vi "uc480_LiveStream_8bitAMb.vi"() -> ()   [LabVIEW 2013]
doc: "Capture_8bit nimmt kontinuierlich Bilder von der Kamera auf und zeigt diese an."
panel:
  out "Row sigma":dbl
  out "Col sigma":dbl
  out "Fits Graphs":cluster{i32[], "Best Gaussian Fit":dbl[]}[](graph)
  out "Row Cent":dbl
  out "Col Cent":dbl
  out "Col 1/e^2 rad":cluster{i32[], dbl[]}(graph)
  out "Row 1/e^2 rad":cluster{i32[], dbl[]}(graph)
  in  "Clip Threshold":dbl
  out "Col Centroid":cluster{i32[], dbl[]}[](graph)
  out "Row Centroid":cluster{i32[], dbl[]}[](graph)
  in  "Clear Charts":bool
  out "Centroid position":cluster{dbl[], dbl[]}(graph)
  out "Staturation":dbl(slide) scale=0.0..255.0
  out "Histogram":dynamicdata(graph)
  out "min value":u8
  out "max value":u8
  out "size(s)":i32[](array[numeric])
  out "output array":u8[][](array[numeric])
  out "error out":errorcluster caption="error"
  in  "Camera ID":u32
  in  "Frame rate":dbl(slide)=30.0 min=4.876716604244694 max=13.962044182888818 step=6.675e-05 scale=4.876716604244694..13.962044182888818 scale format="%^#_3g"
  in  "Pixel clock":i32(slide)=20 min=5 max=43 scale=5.0..43.0
  in  "Exposure time":dbl(slide)=33.21525 min=0.06675 max=71.556 step=0.06675 scale=0.06675..71.556 scale format="%#.3g"
  in  "Edge Filter":i32(ring)=2 items=["High"=1, "Low"=2]
  in  "Edge Filter Enable / Disable":bool
  in  "Blacklevel Offset":i32(slide) min=0 max=255 scale=0.0..255.0
  in  "Blacklevel compensation":bool
  in  "Hotpixel correction":bool
  in  "Master Gain":i32(slide) min=0 max=100 scale=0.0..100.0
  in  "Autogain":bool
  out "Height":i32=480
  out "Width":i32=640
  out "Bits/Pixel":i32=8
  out "FPS":dbl=6.258409738085552
  in  "Stopp":bool
  out "Video":u8[][](graph)
  # "Stop Program here"
  # "2 sigma = 1/e^2 (13.5%) radius\nFWHM = 2.35 sigma"
  # "Image information"
  # "Settings"
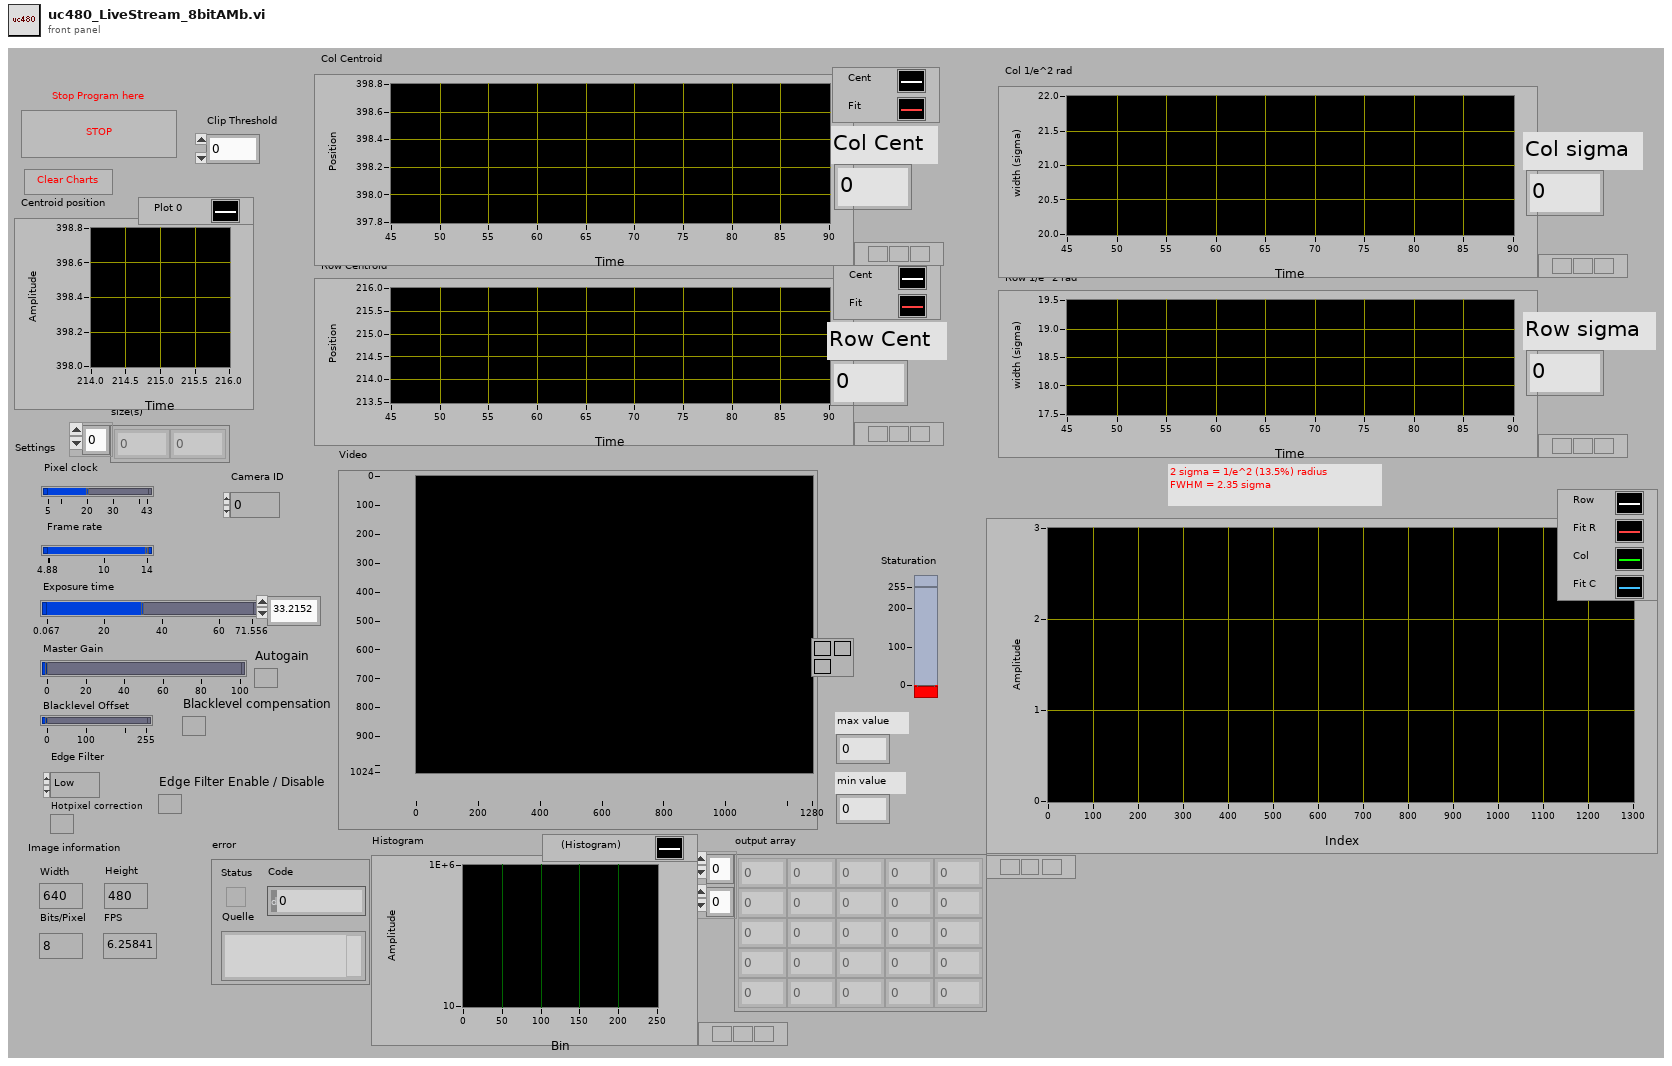
[diagram p1: front panel]
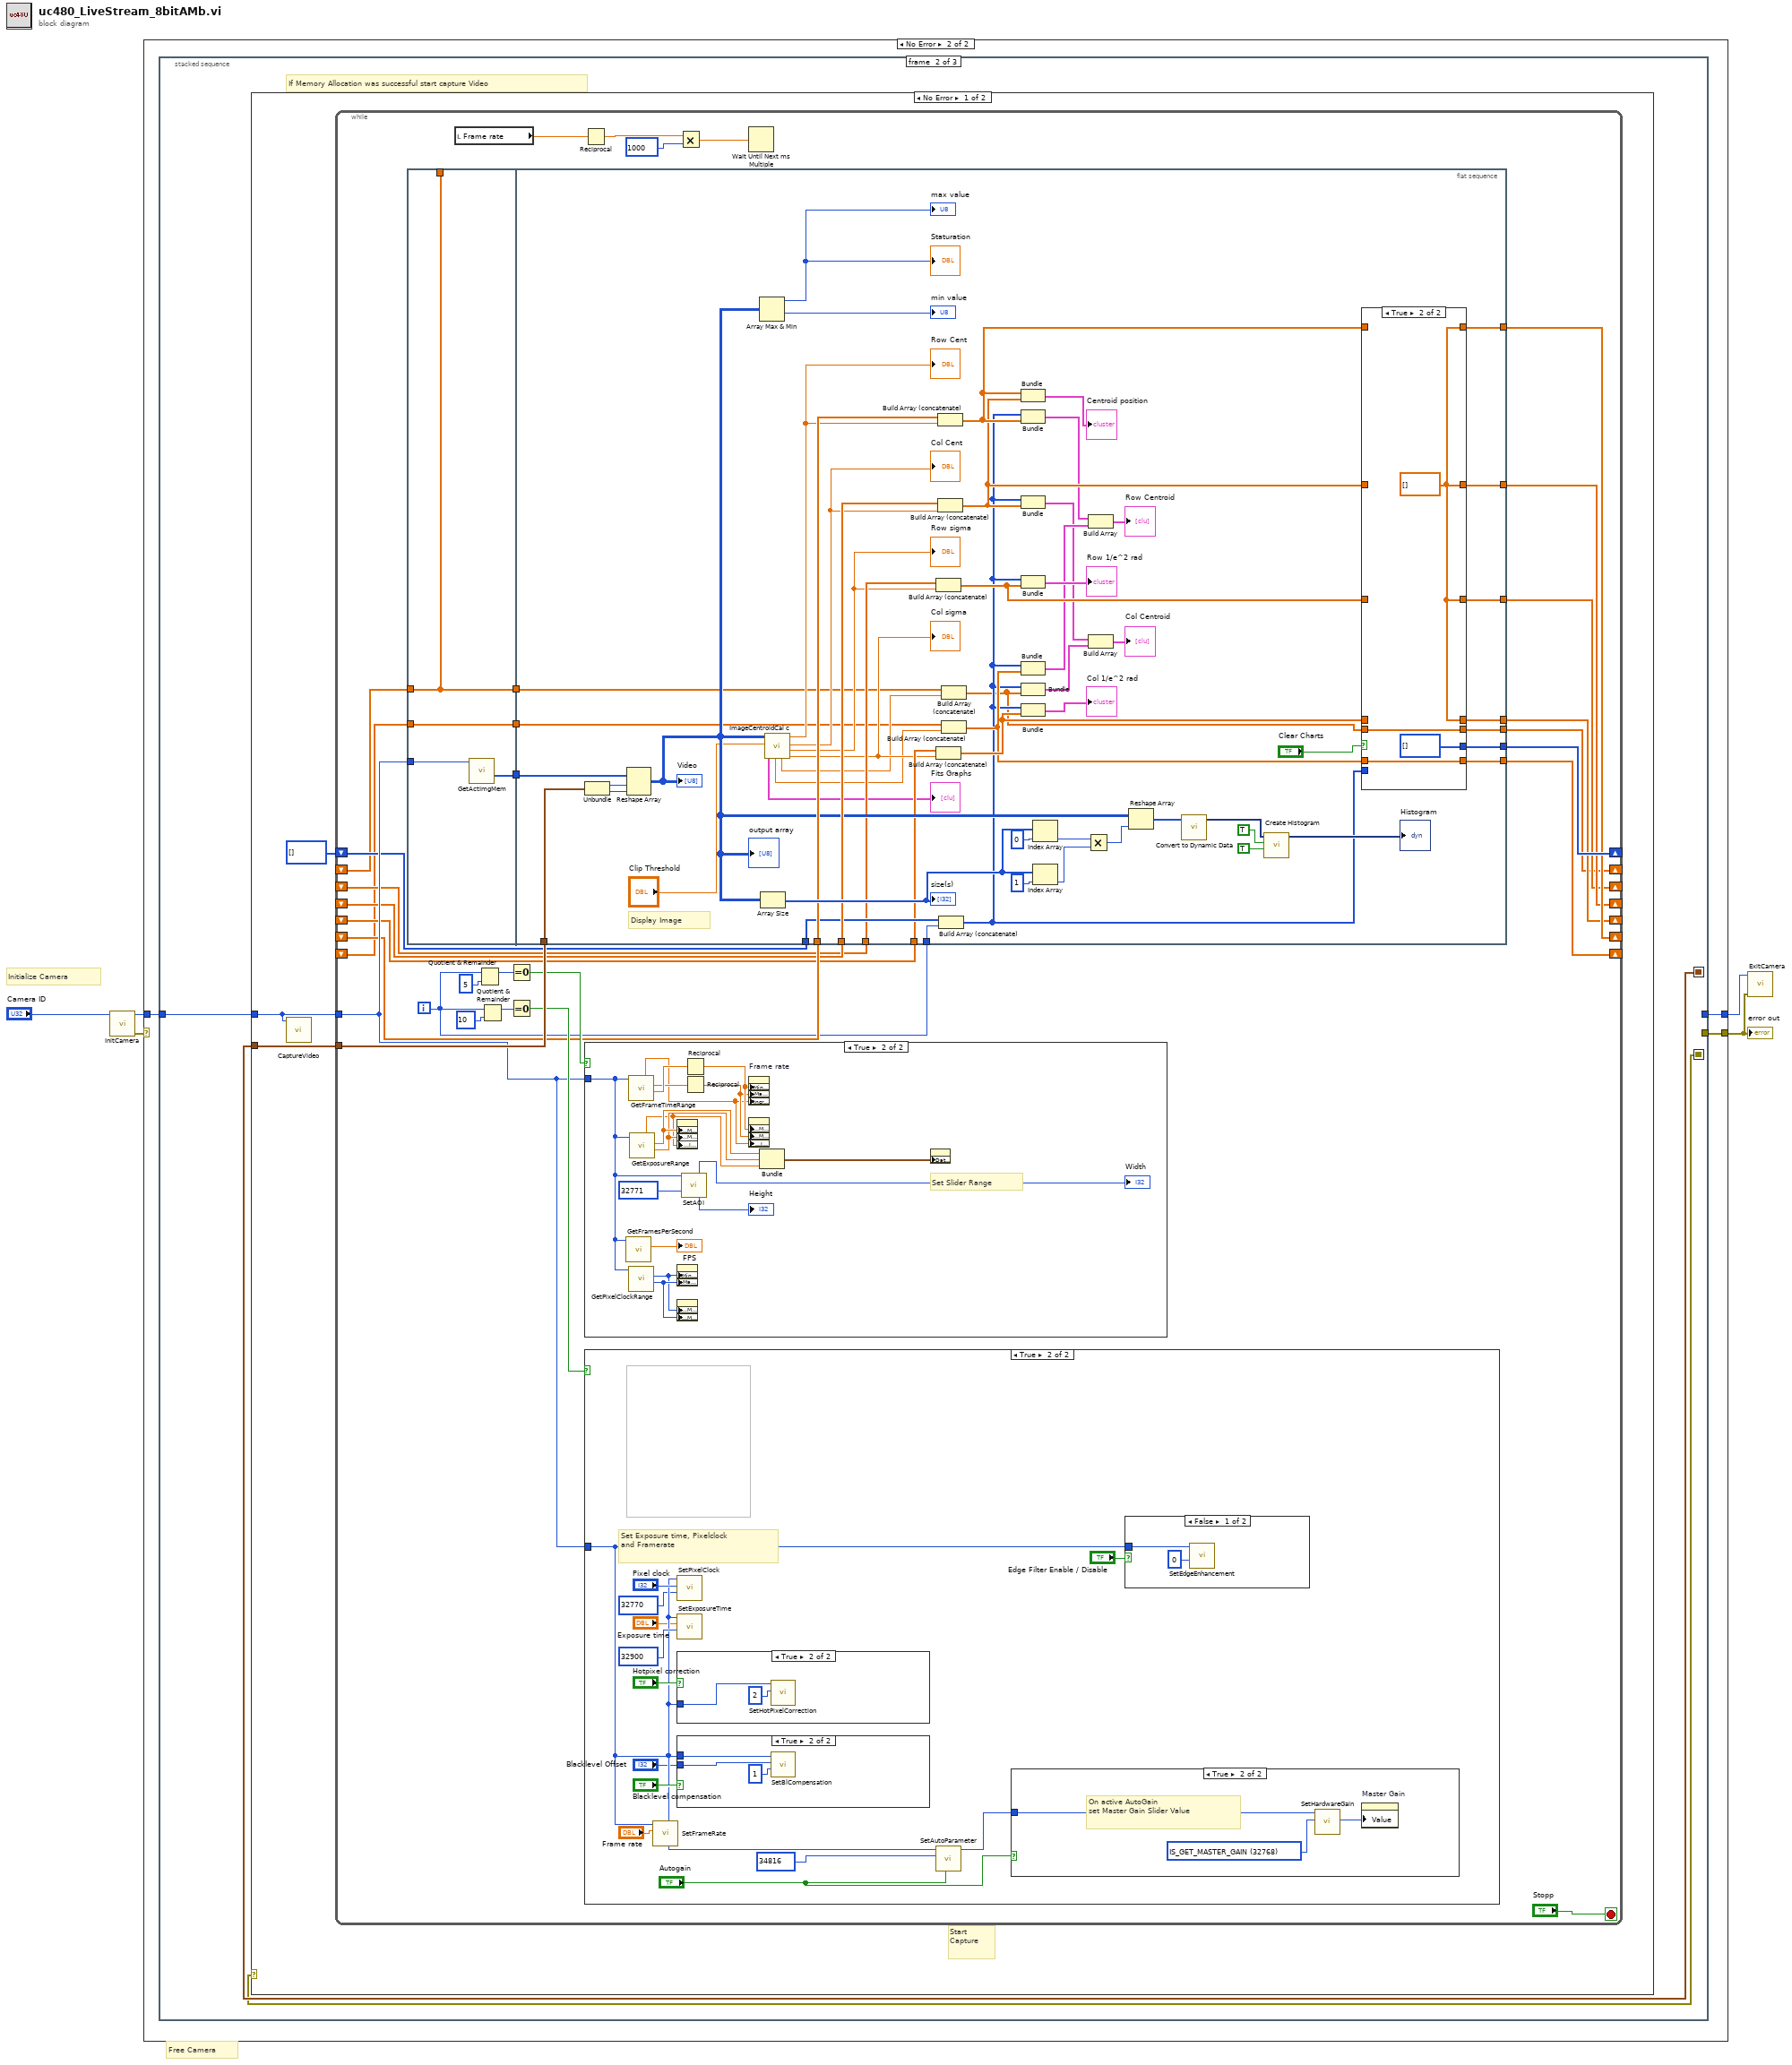
[diagram p0: block diagram]
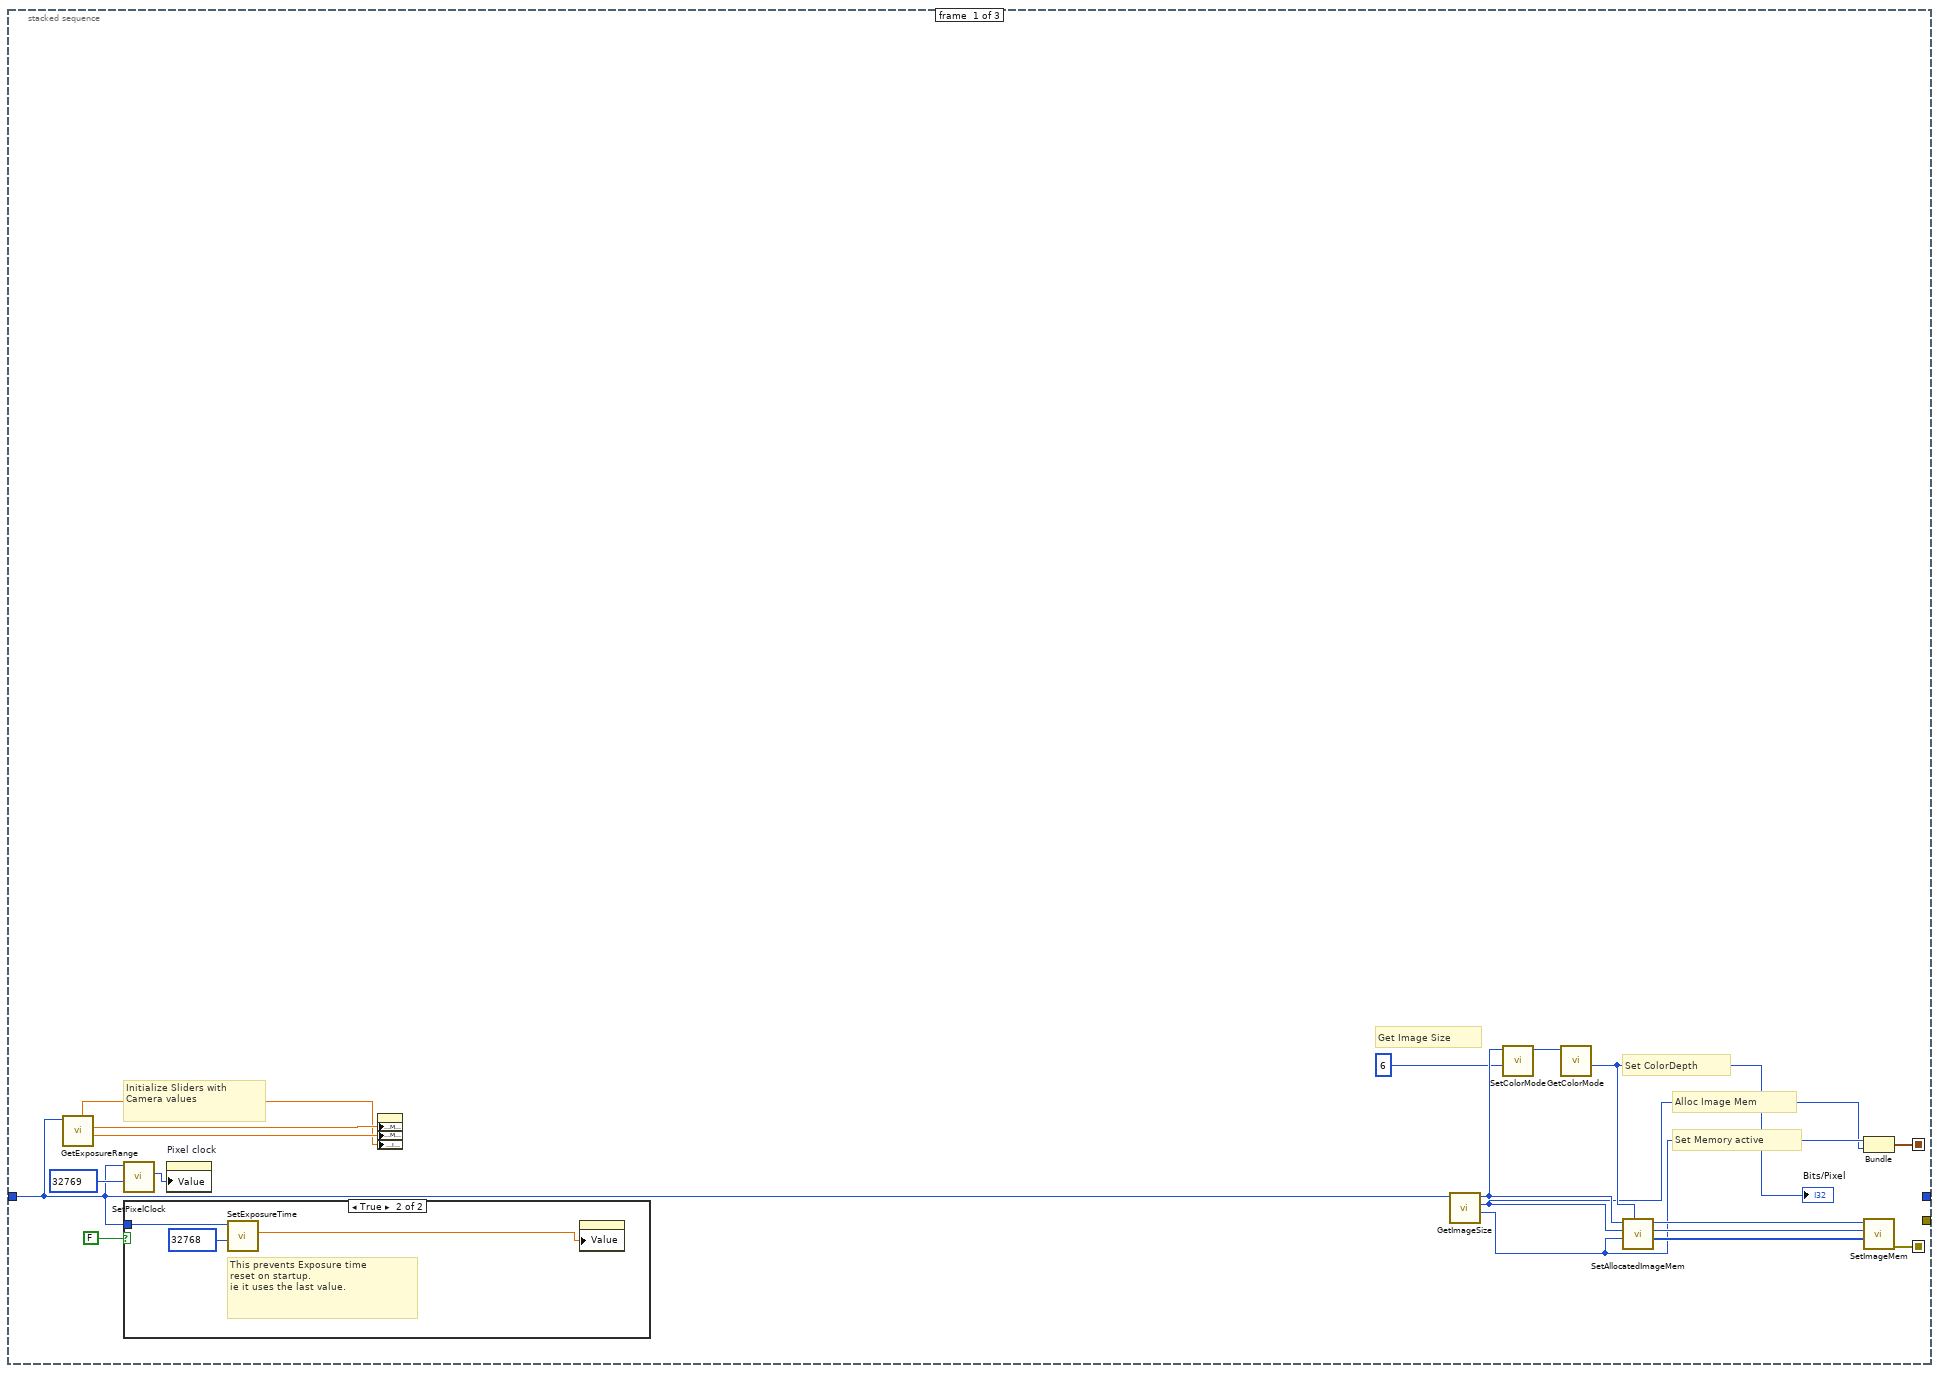
[diagram p3: hidden frame]
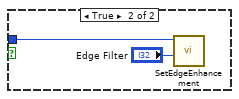
[diagram p6: hidden frame]
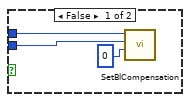
[diagram p7: hidden frame]
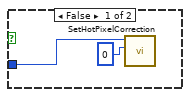
[diagram p8: hidden frame]
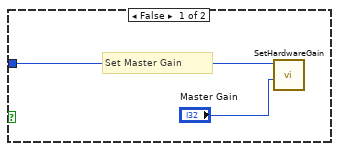
[diagram p9: hidden frame]
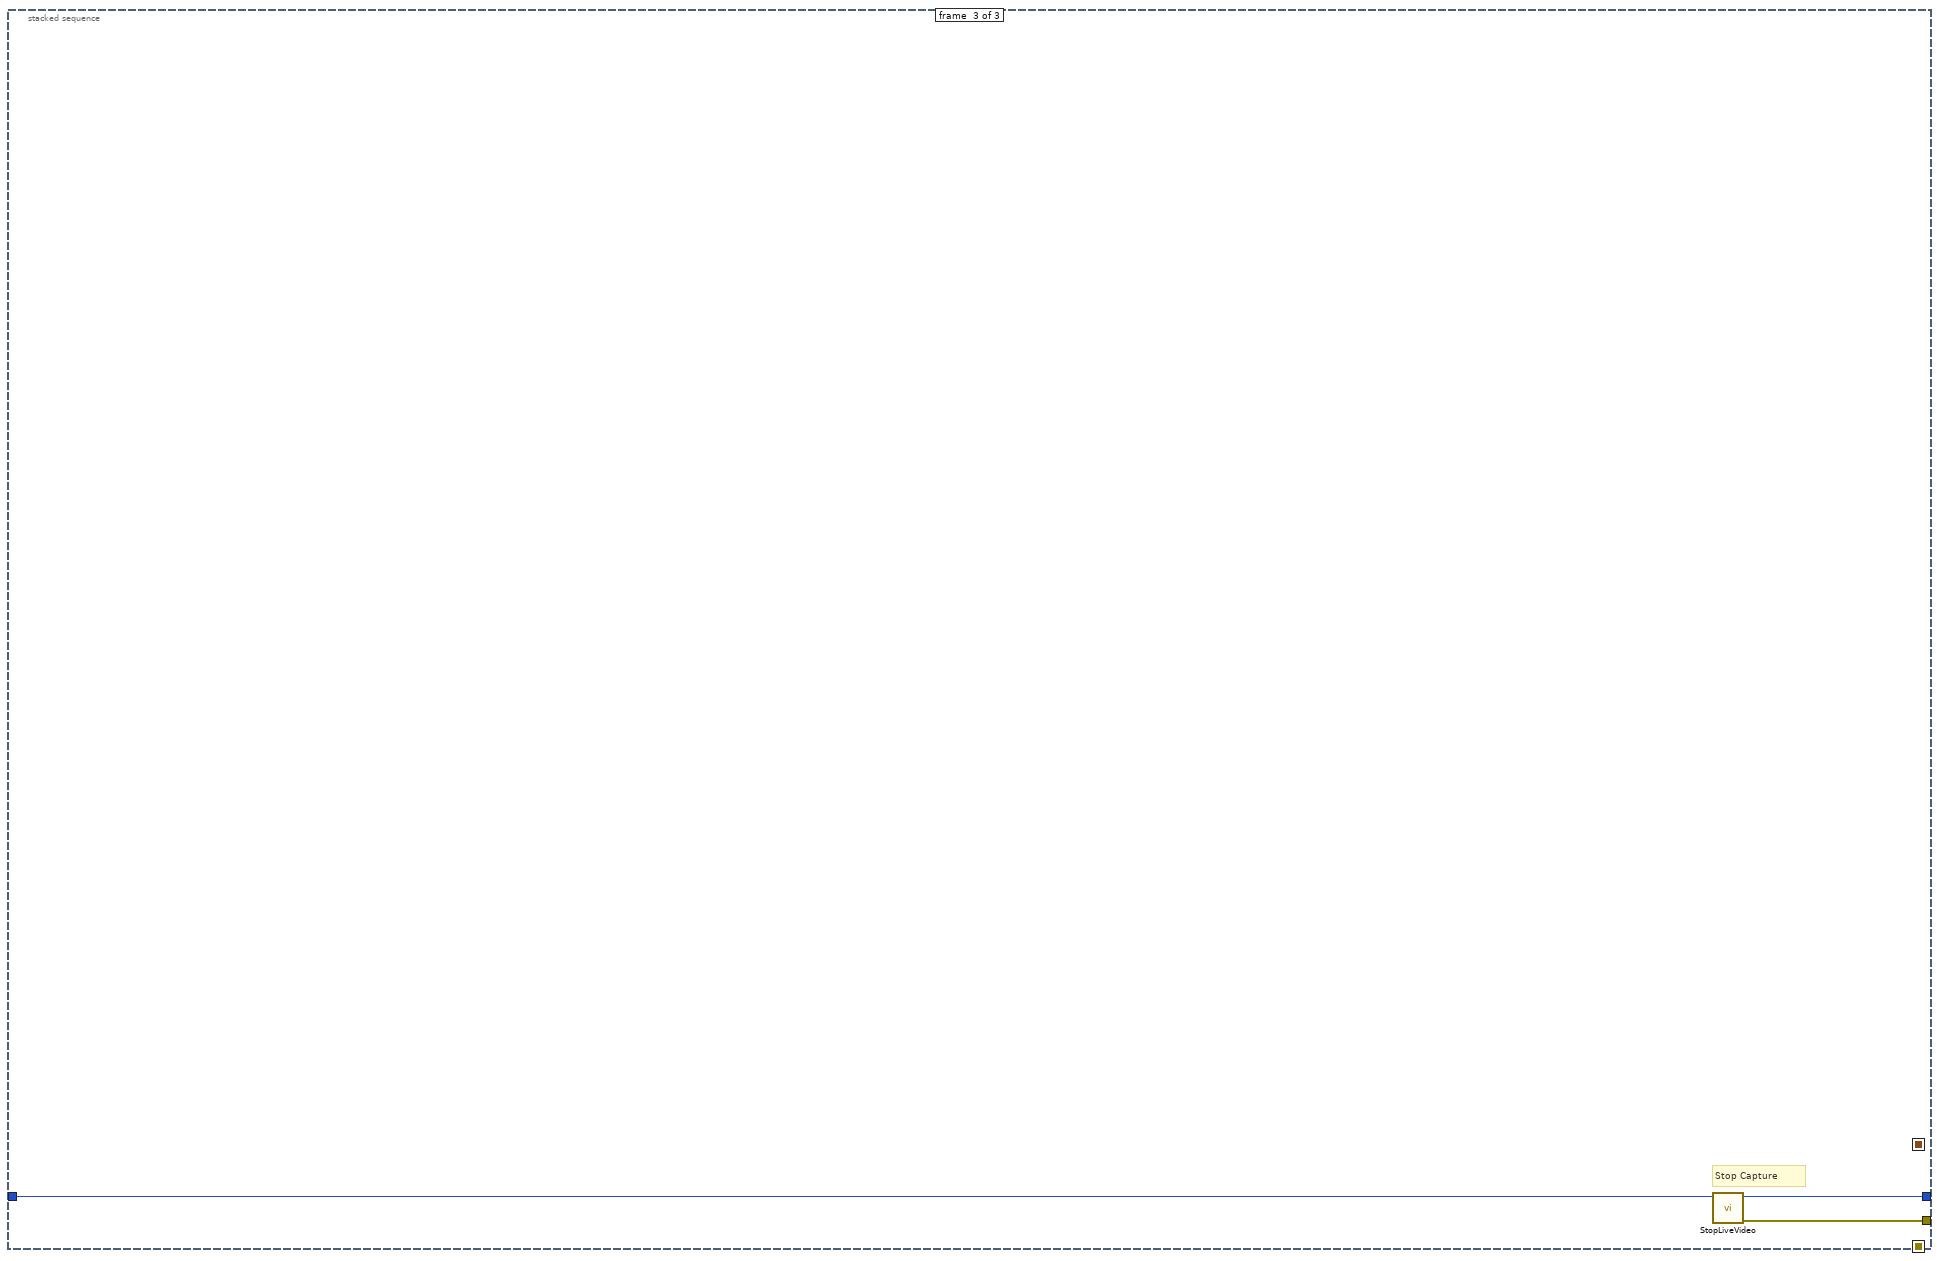
[diagram p13: hidden frame]
diagram:
  # "Free Camera"
  # "Initialize Camera"
  n1 = call "InitCamera.vi"("Camera ID"="Camera ID") -> ("error out"=w2:errorcluster, "Camera Handle Out"=w3:u32)  [unwired: 9 in]
  n2 = case shown="No Error" w2 {
    selector: w2 -> [w6 _]
    tunnel: [w7 w10] -> w5
    tunnel: w3 -> [w7 w9]
    tunnel: [w6 w8] -> w1
    frame Error {
    }
    frame No Error {
      n3 = stacked-sequence {
        seq-local: [w24 _ _] -> [_ w34 _]
        seq-local: [w25 _ _] -> [_ w33 _]
        tunnel: w9 -> [w17 w32 w192]
        tunnel: [_ _ w191] -> w10
        tunnel: [_ _ w190] -> w8
        frame #0 {
          # "Set Memory active"
          # "Alloc Image Mem"
          # "Set ColorDepth"
          # "Initialize Sliders with\nCamera values"
          # "Get Image Size"
          n4 = call "GetExposureRange.vi"("Camera Handle In"=w17) -> ("max"=w21:dbl, "min"=w22:dbl, "intervall"=w20:dbl)  [unwired: 6 in, 2 out]
          n5 = call "SetPixelClock.vi"("Mode"=32769, "Camera Handle In"=w17) -> ("Value"=w19:i32)  [unwired: 7 in, 2 out]
          n6 = case shown="True" FALSE {
            tunnel: w17 -> [_ w29]
            frame False {
            }
            frame True {
              # "This prevents Exposure time\nreset on startup.\nie it uses the last value."
              n7 = call "SetExposureTime.vi"("Mode"=u16 32768, "Camera Handle In"=w29) -> ("new exposure time"=w31:dbl)  [unwired: 7 in, 2 out]
              n8 = property on="Exposure time" class="Slide (strict)"("Value"=w31) -> ()  [unwired: 2 in, 2 out]
            }
          }
          n9 = property on="Pixel clock" class="Slide (strict)"("Value"=w19) -> ()  [unwired: 2 in, 2 out]
          n10 = property on="Exposure time" class="Schieberegler (strikt)"("Scale.Minimum"=w22, "Scale.Maximum"=w21, "Scale.Increment"=w20) -> ()  [unwired: 2 in, 2 out]
          n11 = call "GetImageSize.vi"("Camera Handle In"=w17) -> ("Height"=w13:i32, "Width"=w12:i32, "Camera Handle Out"=w23:u32)  [unwired: 8 in]
          n12 = call "SetColorMode.vi"("Mode"=6, "Camera Handle In"=w23) -> ("Camera Handle Out"=w16:u32)  [unwired: 8 in, 1 out]
          n13 = call "GetColorMode.vi"("Camera Handle In"=w16) -> ("Bits/Pixel"=w14:i32)  [unwired: 8 in, 2 out]
          "Bits/Pixel" <- w14
          n14 = call "SetAllocatedImageMem.vi"("BitsPixel"=w14, "Height"=w13, "Width"=w12, "Camera Handle In"=w23) -> ("Image Memory Out"=w26:u8[], "Memory ID Out"=w27:i32, "Camera Handle Out"=w28:u32)  [unwired: 3 in, 2 out]
          n15 = Bundle("Height"=w13, "Width"=w12) -> (w24:cluster{"Height":i32, "Width":i32})  [unwired: 1 in]
          n16 = call "SetImageMem.vi"("Image Memory In"=w26, "Memory ID In"=w27, "Camera Handle In"=w28) -> ("error out"=w25:errorcluster)  [unwired: 5 in, 3 out]
        }
        frame #1 {
          # "If Memory Allocation was successful start capture Video"
          n17 = case shown="No Error" w33 {
            tunnel: w32 -> [w36 _]
            tunnel: w34 -> [w37 _]
            frame No Error {
              # "Start\nCapture"
              n18 = call "CaptureVideo.vi"("Camera Handle In"=w36) -> ()  [unwired: 9 in, 2 out]
              n19 = while {
                tunnel: w37 -> [w67]
                tunnel: w36 -> [w59]
                shift-right: [w49] -> _
                shift-left: _ -> [w54]
                shift-right: [w48] -> _
                shift-left: _ -> [w53]
                shift-right: [w51] -> _
                shift-left: i32[] [] -> [w50]
                shift-right: [w45] -> _
                shift-left: _ -> [w47]
                shift-right: [w44] -> _
                shift-left: _ -> [w46]
                shift-right: [w39] -> _
                shift-left: _ -> [w42]
                shift-right: [w38] -> _
                shift-left: _ -> [w40]
                i -> [w52]
                stop <- "Stopp" stop-if-true
                n20 = flat-sequence {
                  tunnel: [w119] -> w68
                  tunnel: w59 -> [w120]
                  tunnel: w42 -> [w118]
                  tunnel: [w118] -> w43
                  tunnel: [w117] -> _
                  tunnel: [w117] -> w41
                  tunnel: w40 -> [w117]
                  tunnel: w68 -> [w178]
                  tunnel: w67 -> [w177]
                  tunnel: [w157] -> w49
                  tunnel: w54 -> [w161]
                  tunnel: [w156] -> w48
                  tunnel: w53 -> [w160]
                  tunnel: w52 -> [w159]
                  tunnel: [w154] -> w51
                  tunnel: w50 -> [w158]
                  tunnel: w47 -> [w148]
                  tunnel: w46 -> [w147]
                  tunnel: [w146] -> w45
                  tunnel: [w145] -> w44
                  tunnel: w43 -> [w135]
                  tunnel: w41 -> [w134]
                  tunnel: [w133] -> w39
                  tunnel: [w132] -> w38
                  frame #0 {
                    n21 = call "GetActImgMem.vi"("Camera Handle In"=w120) -> ("Image Memory Out"=w119:u8[])  [unwired: 7 in, 3 out]
                  }
                  frame #1 {
                    # "Display Image"
                    n22 = Unbundle(w177) -> ("Height"=w176:i32, "Width"=w175:i32)
                    n23 = Reshape Array(w178, w176, w175) -> (w152:u8[][])
                    "Video" <- w152
                    "output array" <- w152
                    n24 = Array Max & Min(array=w152) -> (max value=→"max value" →"Staturation":u8, min value=→"min value":u8)  [unwired: 2 out]
                    n25 = Array Size(array=w152) -> (size(s)=w172:i32[])
                    "size(s)" <- w172
                    n26 = call "ImageCentroidCal c.vi"("Clip Threshold"="Clip Threshold", "input array"=w152) -> ("standard dev Col"=w139:dbl, "standard dev Row"=w140:dbl, "Centroid of Cols"=w149:dbl, "Centroid of Rows"=w150:dbl, "fitted center Col"=w136:dbl, "fitted center Row"=w137:dbl, "XY Graph"=→"Fits Graphs":cluster{i32[], "Best Gaussian Fit":dbl[]}[])  [unwired: 1 in, 2 out]
                    "Row Cent" <- w150
                    "Col Cent" <- w149
                    "Row sigma" <- w140
                    "Col sigma" <- w139
                    n27 = Build Array (concatenate)(w148, w140) -> (w144:dbl[])
                    n28 = Build Array (concatenate)(w147, w139) -> (w143:dbl[])
                    n29 = Build Array (concatenate)(w161, w150) -> (w153:dbl[])
                    n30 = Build Array (concatenate)(w160, w149) -> (w130:dbl[])
                    n31 = Build Array (concatenate)(w158, w159) -> (w129:i32[])
                    n32 = Build Array (concatenate)(w134, w136) -> (w124:dbl[])
                    n33 = Build Array (concatenate)(w135, w137) -> (w131:dbl[])
                    n34 = Bundle(w153, w130) -> (→"Centroid position":cluster{dbl[], dbl[]})  [unwired: 1 in]
                    n35 = Bundle(w129, w153) -> (w126:cluster{i32[], dbl[]})  [unwired: 1 in]
                    n36 = Bundle(w129, w130) -> (w122:cluster{i32[], dbl[]})  [unwired: 1 in]
                    n37 = Bundle(w129, w144) -> (→"Row 1/e^2 rad":cluster{i32[], dbl[]})  [unwired: 1 in]
                    n38 = Bundle(w129, w131) -> (w127:cluster{i32[], dbl[]})  [unwired: 1 in]
                    n39 = Bundle(w129, w124) -> (w123:cluster{i32[], dbl[]})  [unwired: 1 in]
                    n40 = Bundle(w129, w143) -> (→"Col 1/e^2 rad":cluster{i32[], dbl[]})  [unwired: 1 in]
                    n41 = Index Array(array=w172, index=0) -> (element=w170:i32)
                    n42 = Index Array(array=w172, index=1) -> (element=w169:i32)
                    n43 = Multiply(x=w170, y=w169) -> (x*y=w168:i32)
                    n44 = Build Array(w126, w127) -> (→"Row Centroid":cluster{i32[], dbl[]}[])
                    n45 = Build Array(w122, w123) -> (→"Col Centroid":cluster{i32[], dbl[]}[])
                    n46 = Reshape Array(w152, w168) -> (w167:u8[])
                    n47 = call "Convert to Dynamic Data"("Array"=w167) -> ("Dynamic Data Type"=w166:dynamicdata)  [unwired: 3 in]
                    n48 = call "Create Histogram"("Reset"=TRUE, "Enable"=TRUE, "Signal"=w166) -> ("Histogram"=→"Histogram":dynamicdata)  [unwired: 7 in, 1 out]
                    n49 = case shown="True" "Clear Charts" {
                      tunnel: w153 -> [w185 _]
                      tunnel: w130 -> [w184 _]
                      tunnel: [w185 w188] -> w157
                      tunnel: [w184 w188] -> w156
                      tunnel: w129 -> [w183 _]
                      tunnel: [w183 i32[] []] -> w154
                      tunnel: w144 -> [w182 _]
                      tunnel: [w182 w188] -> w146
                      tunnel: w143 -> [w181 _]
                      tunnel: [w181 w188] -> w145
                      tunnel: w131 -> [w180 w187]
                      tunnel: [w180 w187] -> w133
                      tunnel: w124 -> [w179 w186]
                      tunnel: [w179 w186] -> w132
                      frame False {
                      }
                      frame True {
                        w188 = dbl[] []
                      }
                    }
                  }
                }
                n50 = local read "Frame rate"() -> (w58:dbl)
                n51 = Quotient & Remainder(x=w52, y=5) -> (x-y*floor(x/y)=w65:i32)  [unwired: 1 out]
                n52 = Quotient & Remainder(x=w52, y=10) -> (x-y*floor(x/y)=w62:i32)  [unwired: 1 out]
                n53 = Equal To 0?(x=w65) -> (x = 0?=w64:bool)
                n54 = Equal To 0?(x=w62) -> (x = 0?=w60:bool)
                n55 = Reciprocal(x=w58) -> (1/x=w57:dbl)
                n56 = case shown="True" w64 {
                  tunnel: w59 -> [_ w103]
                  frame False {
                  }
                  frame True {
                    # "Set Slider Range"
                    n57 = call "GetFramesPerSecond.vi"("Camera Handle In"=w103) -> ("FPS"=→"FPS":dbl)  [unwired: 8 in, 2 out]
                    n58 = call "GetFrameTimeRange.vi"("Camera Handle In"=w103) -> ("max"=w109:dbl, "min"=w108:dbl, "interval"=w105:dbl)  [unwired: 6 in, 2 out]
                    n59 = call "GetPixelClockRange.vi"("Camera Handle In"=w103) -> ("Max"=w111:i32, "Min"=w110:i32)  [unwired: 7 in, 2 out]
                    n60 = call "GetExposureRange.vi"("Camera Handle In"=w103) -> ("max"=w113:dbl, "min"=w114:dbl, "intervall"=w112:dbl)  [unwired: 6 in, 2 out]
                    n61 = property on="Exposure time" class="Schieberegler (strikt)"("Scale.Minimum"=w114, "Scale.Maximum"=w113, "Scale.Increment"=w112) -> ()  [unwired: 2 in, 2 out]
                    n62 = property on="Pixel clock" class="Schieberegler (strikt)"("Minimum"=w110, "Maximum"=w111) -> ()  [unwired: 2 in, 2 out]
                    n63 = property on="Pixel clock" class="Schieberegler (strikt)"("Scale.Minimum"=w110, "Scale.Maximum"=w111) -> ()  [unwired: 2 in, 2 out]
                    n64 = call "SetAOI.vi"("Camera Handle In"=w103, "Mode"=32771) -> ("Width Out"=→"Width":i32, "Height Out"=→"Height":i32)  [unwired: 8 in, 4 out]
                    n65 = Reciprocal(x=w109) -> (1/x=w107:dbl)
                    n66 = Reciprocal(x=w108) -> (1/x=w106:dbl)
                    n67 = property on="Frame rate" class="Schieberegler (strikt)"("Minimum"=w107, "Maximum"=w106, "Increment"=w105) -> ()  [unwired: 2 in, 2 out]
                    n68 = property on="Frame rate" class="Schieberegler (strikt)"("Scale.Minimum"=w107, "Scale.Maximum"=w106, "Scale.Increment"=w105) -> ()  [unwired: 2 in, 2 out]
                    n69 = Bundle("min"=w114, "max"=w113, "intervall"=w112) -> (w115:cluster{"min":dbl, "max":dbl, "intervall":dbl})  [unwired: 1 in]
                    n70 = property on="Exposure time" class="Schieberegler (strikt)"("Data Range"=w115) -> ()  [unwired: 2 in, 2 out]
                  }
                }
                n71 = case shown="True" w60 {
                  tunnel: w59 -> [_ w72]
                  frame False {
                  }
                  frame True {
                    # "Set Exposure time, Pixelclock\nand Framerate"
                    n72 = call "SetFrameRate.vi"("FPS"="Frame rate", "Camera Handle In"=w72) -> ()  [unwired: 7 in, 3 out]
                    n73 = call "SetPixelClock.vi"("Mode"=32770, "Pixel Clock"="Pixel clock", "Camera Handle In"=w72) -> ()  [unwired: 6 in, 3 out]
                    n74 = call "SetExposureTime.vi"("Mode"=u16 32900, "Exposure Time"="Exposure time", "Camera Handle In"=w72) -> ()  [unwired: 6 in, 3 out]
                    n75 = case shown="True" "Hotpixel correction" {
                      tunnel: w72 -> [w93 w95]
                      frame False {
                        n76 = call "SetHotPixelCorrection.vi"("Mode"=0, "Camera Handle In"=w93) -> ()  [unwired: 7 in, 3 out]
                      }
                      frame True {
                        n77 = call "SetHotPixelCorrection.vi"("Mode"=2, "Camera Handle In"=w95) -> ()  [unwired: 7 in, 3 out]
                      }
                    }
                    n78 = case shown="True" "Blacklevel compensation" {
                      tunnel: w72 -> [w88 w91]
                      tunnel: "Blacklevel Offset" -> [w86 w89]
                      frame False {
                        n79 = call "SetBlCompensation.vi"("Mode"=0, "offset"=w86, "Camera Handle In"=w88) -> ()  [unwired: 6 in, 3 out]
                      }
                      frame True {
                        n80 = call "SetBlCompensation.vi"("Mode"=1, "offset"=w89, "Camera Handle In"=w91) -> ()  [unwired: 6 in, 3 out]
                      }
                    }
                    n81 = call "SetAutoParameter.vi"("enable"="Autogain", "Param"=34816, "Camera Handle In"=w72) -> ("Camera Handle Out"=w80:u32)  [unwired: 6 in, 2 out]
                    n82 = case shown="True" "Autogain" {
                      tunnel: w80 -> [w96 w99]
                      frame False {
                        # "Set Master Gain"
                        n83 = call "SetHardwareGain.vi"("Master Gain"="Master Gain", "Camera Handle In"=w96) -> ()  [unwired: 7 in, 3 out]
                      }
                      frame True {
                        w98 = 32768 items=["IS_GET_MASTER_GAIN"=32768]
                        # "On active AutoGain\nset Master Gain Slider Value"
                        n84 = call "SetHardwareGain.vi"("Mode"=w98, "Camera Handle In"=w99) -> ("Value"=w100:i32)  [unwired: 7 in, 2 out]
                        n85 = property on="Master Gain" class="Slide (strict)"("Value"=w100) -> ()  [unwired: 2 in, 2 out]
                      }
                    }
                    n86 = case shown="False" "Edge Filter Enable / Disable" {
                      tunnel: w72 -> [w82 w85]
                      frame False {
                        n87 = call "SetEdgeEnhancement.vi"("Mode"=0, "Camera Handle In"=w82) -> ()  [unwired: 8 in, 2 out]
                      }
                      frame True {
                        n88 = call "SetEdgeEnhancement.vi"("Mode"="Edge Filter", "Camera Handle In"=w85) -> ()  [unwired: 8 in, 2 out]
                      }
                    }
                  }
                }
                n89 = Multiply(x=w57, y=1000) -> (x*y=w55:dbl)
                n90 = Wait Until Next ms Multiple(millisecond multiple=w55) -> ()  [unwired: 1 out]
              }
            }
            frame Error {
            }
          }
        }
        frame #2 {
          # "Stop Capture"
          n91 = call "StopLiveVideo.vi"("Camera Handle In"=w192) -> ("error out"=w190:errorcluster, "Camera Handle Out"=w191:u32)  [unwired: 9 in]
        }
      }
    }
  }
  "error out" <- w1
  n92 = call "ExitCamera.vi"("error in"=w1, "Camera Handle In"=w5) -> ()  [unwired: 9 in, 1 out]
